vi "Pump Status Gat.vi"(8 "error in (no error)":errorcluster, 10 "Enum in":refnum<vi>, 11 "VICI Settings in":T1) -> (0 "error out":errorcluster, 1 "Connection Error":bool, 2 "Pump On?":enum16{"Off", "On", "Not Initialized"}(ring), 3 "VICI Settings out":T1, 4 "microliters/min":dbl)   [LabVIEW 2018, in "VICI M6 M50 Party Mode.lvlib"]
uses:
  VICI M6 M50 Party Mode.lvlib
  \\smbgbl.drmvfs102.pfizer.com\FAST_Team/Software/LabVIEW/Third Party Drivers/Third Party Drivers/VICI/Global FIA milliGAT.lvlib
  Settings Cluster.ctl
panel:
  out "moving":bool
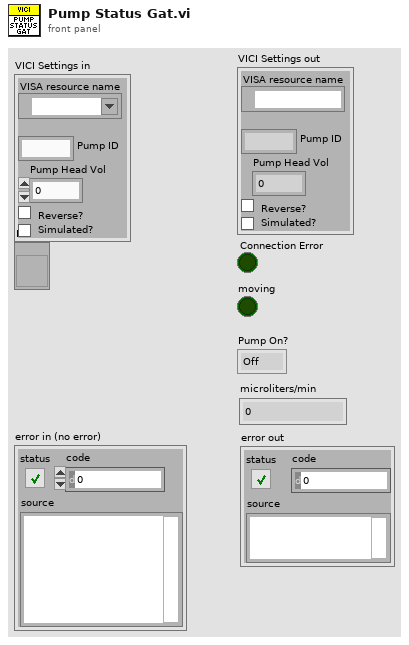
[diagram p1: front panel]
types:
  T1 = typedef "VICI M6 M50 Party Mode.lvlib/Settings Cluster.ctl" = cluster{"VISA resource name":refnum<visa-resource-name>, "Pump ID":string, "Pump Head Vol":dbl, "Reverse?":bool, "Simulated?":bool}
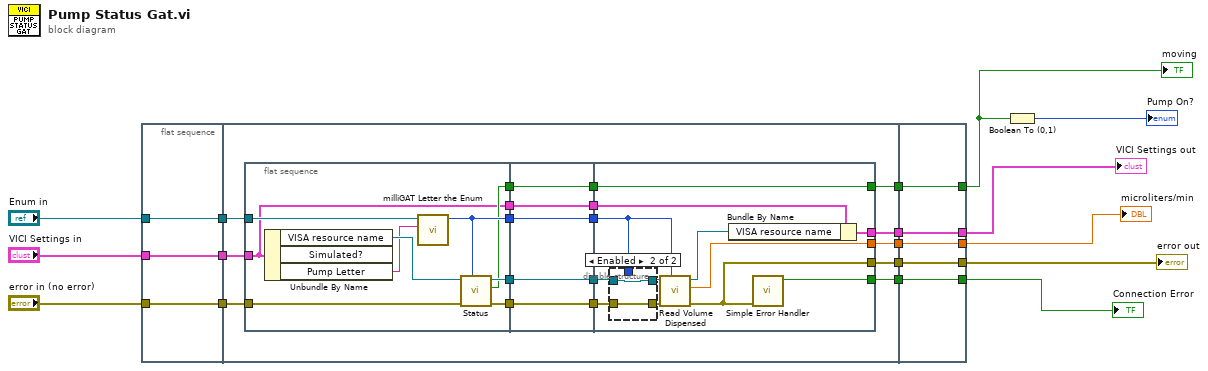
[diagram p0: block diagram]
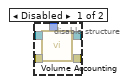
[diagram p2: hidden frame]
diagram:
  n1 = flat-sequence {
    tunnel: "error in (no error)" -> [w18]
    tunnel: "Enum in" -> [w19]
    tunnel: "VICI Settings in" -> [w20]
    tunnel: [w20] -> w4
    tunnel: [w19] -> w3
    tunnel: [w18] -> w2
    tunnel: [w26] -> w9
    tunnel: [w21] -> w8
    tunnel: [w25] -> w7
    tunnel: [w24] -> w6
    tunnel: [w35] -> w5
    tunnel: w4 -> [w37]
    tunnel: w3 -> [w38]
    tunnel: w2 -> [w36]
    tunnel: [w72] -> w10
    tunnel: [w73] -> w1
    tunnel: [w74] -> w11
    tunnel: [w75] -> w12
    tunnel: [w76] -> w13
    tunnel: w9 -> [w76]
    tunnel: w8 -> [w75]
    tunnel: w7 -> [w74]
    tunnel: w6 -> [w73]
    tunnel: w5 -> [w72]
    frame #0 {
    }
    frame #1 {
      n2 = flat-sequence {
        tunnel: w38 -> [w42]
        tunnel: w37 -> [w39]
        tunnel: w36 -> [w41]
        tunnel: [w47] -> w34
        tunnel: [w46] -> w33
        tunnel: [w43] -> w32
        tunnel: [w40] -> w31
        tunnel: [w39] -> w23
        tunnel: w34 -> [w52]
        tunnel: w33 -> [w51]
        tunnel: w32 -> [w50]
        tunnel: w31 -> [w49]
        tunnel: [w52] -> w30
        tunnel: [w51] -> w29
        tunnel: [w50] -> w28
        tunnel: [w49] -> w27
        tunnel: w23 -> [w48]
        tunnel: [w48] -> w22
        tunnel: [w64] -> w35
        tunnel: w30 -> [w54]
        tunnel: w29 -> [w57]
        tunnel: w28 -> [w55]
        tunnel: w27 -> [w64]
        tunnel: [w62] -> w26
        tunnel: [w61] -> w25
        tunnel: [w60] -> w24
        tunnel: [w59] -> w21
        tunnel: w22 -> [w58]
        frame #0 {
          n3 = Unbundle By Name(w39) -> ("VISA resource name"=w45:refnum<visa-resource-name>, "Pump Letter"=w44:string)  [unwired: 1 out]
          n4 = call "milliGAT Letter the Enum.vi"("Pump Letter"=w44, "Enum in"=w42) -> ("Numeric"=w43:i32)  [unwired: 9 in]
          n5 = call "Status.vi"("Pump ID (0:A)"=w43, "error in (no error)"=w41, "VISA resource in"=w45) -> ("error out"=w47:errorcluster, "moving"=w40:bool, "VISA resource out"=w46:refnum<visa-resource-name>)  [unwired: 6 in]
        }
        frame #1 {
        }
        frame #2 {
          n6 = disable-structure shown="Enabled" {
            disable-tunnel: w57 -> [w69 w71]
            disable-tunnel: [w68 w71] -> w56
            disable-tunnel: w55 -> [w67 _]
            disable-tunnel: w54 -> [w66 w70]
            disable-tunnel: [w65 w70] -> w53
            frame Disabled {
              n7 = call "Volume Accounting.vi"("Pump ID (0:A)"=w67, "error in (no error)"=w66, "VISA resource in"=w69) -> ("error out"=w65:errorcluster, "VISA resource out"=w68:refnum<visa-resource-name>)  [unwired: 7 in]
            }
            frame Enabled {
            }
          }
          n8 = call "Read Volume Dispensed.vi"("Pump ID (0:A)"=w55, "error in (no error)"=w53, "VISA resource in"=w56) -> ("error out"=w61:errorcluster, "microliters"=w60:dbl, "VISA resource out"=w63:refnum<visa-resource-name>)  [unwired: 6 in]
          n9 = Bundle By Name(cluster=w58, "VISA resource name"=w63) -> (w59:T1)
          n10 = call <vilib>:"Simple Error Handler.vi"("error in (no error)"=w61) -> ("error?"=w62:bool)  [unwired: 4 in, 4 out]
        }
      }
    }
    frame #2 {
    }
  }
  n11 = Boolean To (0,1)(Boolean=w10) -> (0, 1=→"Pump On?":i16)
  "moving" <- w10
  "error out" <- w11
  "microliters/min" <- w1
  "VICI Settings out" <- w12
  "Connection Error" <- w13
